vi "Fan Temperature Initialization.vi"(8 "error in":errorcluster) -> (0 "error out":errorcluster, 3 "DAQmx Task":refnum<k21>)   [LabVIEW 2020]
uses:
  <vilib>/DAQmx/create/channels.llb/DAQmx Create Channel (AI-Temperature-Thermocouple).vi
  <vilib>/DAQmx/configure/timing.llb/DAQmx Timing (Sample Clock).vi
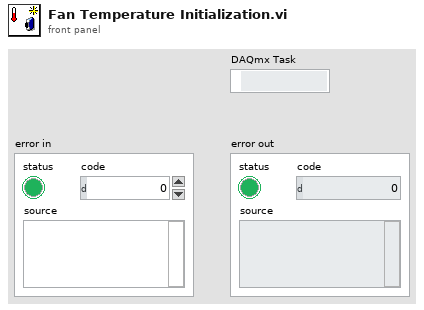
[diagram p1: front panel]
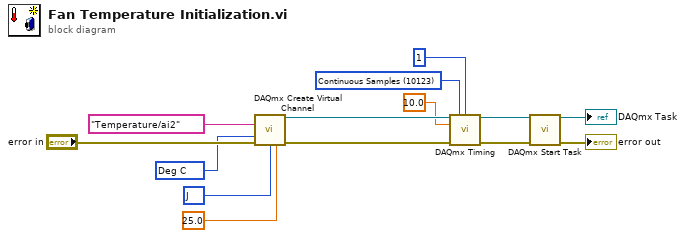
[diagram p0: block diagram]
diagram:
  w1 = 10143 items=["Deg C"=10143, "Deg F"=10144, "Kelvins"=10325, "Deg R"=10145, "From Custom Scale"=10065] ("units")
  w3 = 10072 items=["J"=10072, "K"=10073, "N"=10077, "R"=10082, "S"=10085, "T"=10086, "B"=10047, "E"=10055] ("thermocouple type")
  w10 = 10123 items=["Finite Samples"=10178, "Continuous Samples"=10123, "Hardware Timed Single Point"=12522] ("sample mode")
  n1 = call-poly <vilib>:"DAQmx Create Virtual Channel.vi"("physical channels"=tag "Temperature/ai2", "units"=w1, "error in"="error in", "thermocouple type"=w3, "cjc value"=25.0) -> ("task out"=w14:refnum<k21>, "error out"=w13:errorcluster)  [unwired: 9 in]
  n2 = call-poly <vilib>:"DAQmx Timing.vi"("task/channels in"=w14, "sample mode"=w10, "samples per channel"=1, "rate"=10.0, "error in"=w13) -> ("task out"=w12:refnum<k21>, "error out"=w11:errorcluster)  [unwired: 9 in]
  n3 = call <vilib>:"DAQmx Start Task.vi"("task/channels in"=w12, "error in"=w11) -> ("task out"=→"DAQmx Task":refnum<k21>, "error out"=→"error out":errorcluster)  [unwired: 12 in]
